vi "Queue Self.vi"(9 "Priority?":bool, 10 "Msg":refnum<class "Msg.lvclass">, 11 "jettl Queue Actor in":refnum<class "jettl Queue Actor.lvclass">) -> (3 "jettl Queue Actor out":refnum<class "jettl Queue Actor.lvclass">)   [LabVIEW 2021, in "jettl.lvlib" / "jettl Queue Actor.lvclass"]
uses:
  jettl Queue Actor.lvclass
  Actor/Msg/Msg.lvclass
  jettl Queue Actor.lvclass/jettl Queue Actor.ctl
  jettl.lvlib
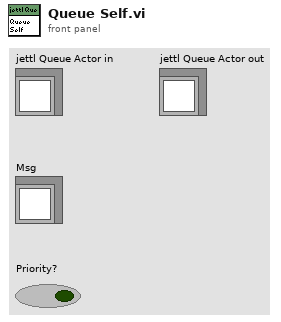
[diagram p1: front panel]
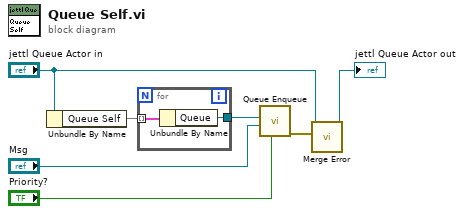
[diagram p0: block diagram]
diagram:
  n1 = Unbundle By Name("jettl Queue Actor in") -> ("Queue Self"=w1:map{string, refnum<data-value>})
  n2 = for {
    tunnel: [w8] -> w2
    tunnel: w1 -> [w9] mode=indexing
    n3 = Unbundle By Name(w9) -> ("Queue"=w8:refnum<data-value>)
  }
  n4 = call "Queue Enqueue.vi"("Priority?"="Priority?", "Msg"="Msg", "Queue"=w2) -> ("error out"=w3:errorcluster)  [unwired: 8 in]
  n5 = call-dynamic "Merge Error.vi"("Error"=w3, "jettl Queue Actor in"="jettl Queue Actor in") -> ("jettl Queue Actor out"=→"jettl Queue Actor out":refnum<class "jettl Queue Actor.lvclass">)  [unwired: 9 in]
